vi "VGC50 Read Pressures.vi"(8 "error in (no error)":errorcluster, 11 "VGC50 In":T1={"serial settings"={"port"="", "baud rate"=115200}, "device information"={"type"="", "model number"="", "serial number"="", "firmware version"="", "hardware version"=""}, "VGC"=refnum, "Backing SP"={"mode"=0, "thresholds"={"lower"=0.0, "upper"=0.0}, "on"=FALSE}, "Chamber SP"={"mode"=1, "thresholds"={"lower"=0.0, "upper"=0.0}, "on"=FALSE}} {"Chamber SP"."thresholds"."upper" format="%#_5p"; "Chamber SP"."thresholds"."lower" format="%#_5p"; "Chamber SP"."mode" items=["off", "on", "channel 1", "channel 2", "channel 3"]; "Backing SP"."thresholds"."upper" format="%#_5p"; "Backing SP"."thresholds"."lower" format="%#_5p"; "Backing SP"."mode" items=["off", "on", "channel 1", "channel 2", "channel 3"]; "serial settings"."baud rate" items=["9600"=9600, "19200"=19200, "38400"=38400, "57600"=57600, "115200"=115200]}) -> (0 "error out":errorcluster, 1 "Chamber Pressure":dbl, 2 "Backing Pressure":dbl, 3 "VGC50 Out":T1={"serial settings"={"port"="", "baud rate"=115200}, "device information"={"type"="", "model number"="", "serial number"="", "firmware version"="", "hardware version"=""}, "VGC"=refnum, "Backing SP"={"mode"=0, "thresholds"={"lower"=0.0, "upper"=0.0}, "on"=FALSE}, "Chamber SP"={"mode"=1, "thresholds"={"lower"=0.0, "upper"=0.0}, "on"=FALSE}} {"Chamber SP"."thresholds"."upper" format="%#_5p"; "Chamber SP"."thresholds"."lower" format="%#_5p"; "Chamber SP"."mode" items=["off", "on", "channel 1", "channel 2", "channel 3"]; "Backing SP"."thresholds"."upper" format="%#_5p"; "Backing SP"."thresholds"."lower" format="%#_5p"; "Backing SP"."mode" items=["off", "on", "channel 1", "channel 2", "channel 3"]; "serial settings"."baud rate" items=["9600"=9600, "19200"=19200, "38400"=38400, "57600"=57600, "115200"=115200]}, 4 "Waveform Chart":waveform(dbl)[](graph))   [LabVIEW 2024]
uses:
  controls/VGC50.ctl
  <instrlib>/PL Inficon VGC/PL Inficon VGC.lvclass
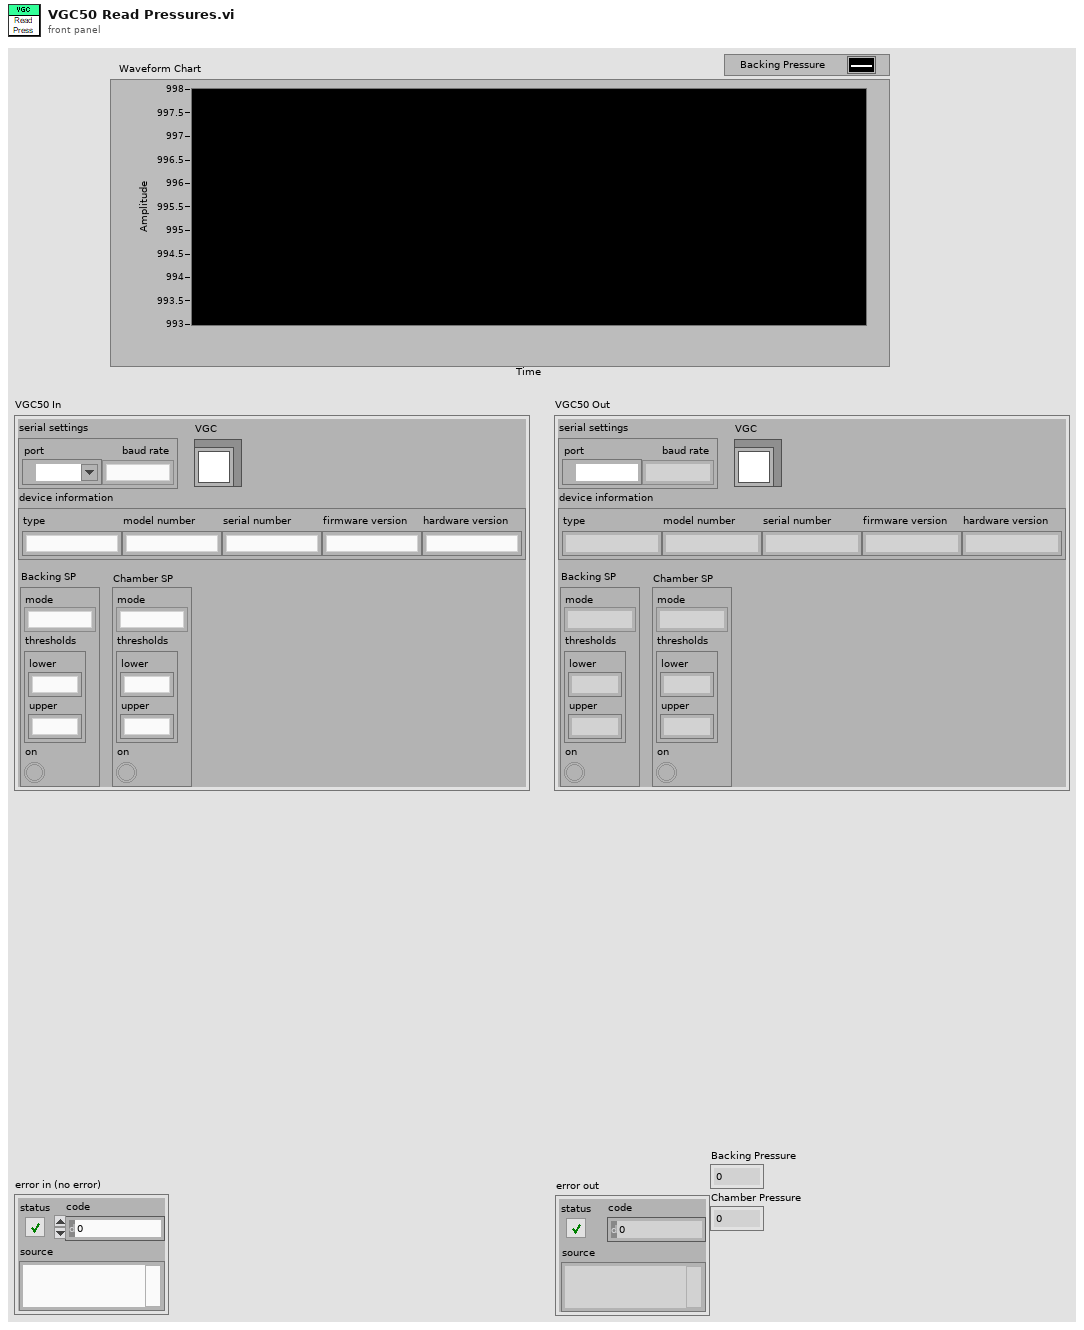
[diagram p1: front panel]
types:
  T1 = typedef "VGC50.ctl" = cluster{"serial settings":cluster{"port":refnum<visa-resource-name>, "baud rate":u32}, "device information":cluster{"type":string, "model number":string, "serial number":string, "firmware version":string, "hardware version":string}, "VGC":refnum<class "PL Inficon VGC.lvclass">, "Backing SP":cluster{"mode":u16, "thresholds":cluster{"lower":dbl, "upper":dbl}, "on":bool}, "Chamber SP":cluster{"mode":u16, "thresholds":cluster{"lower":dbl, "upper":dbl}, "on":bool}}
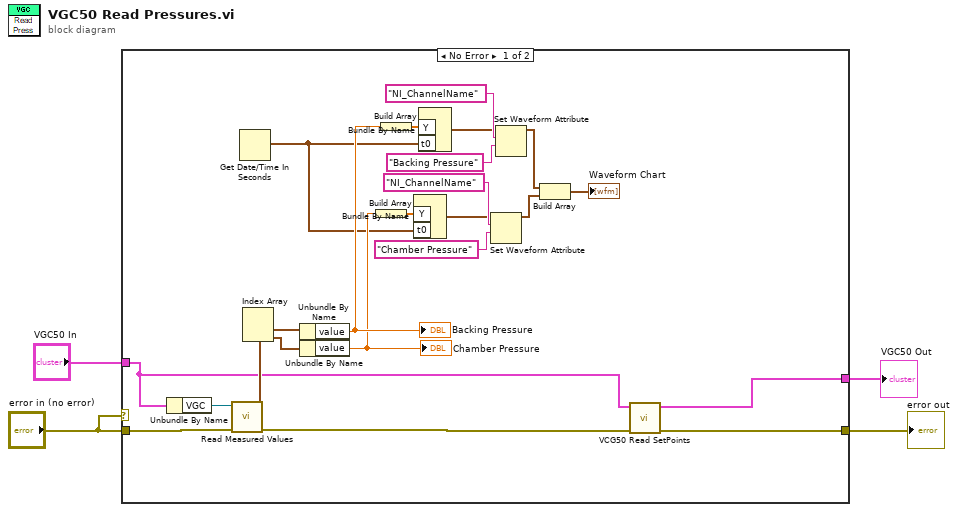
[diagram p0: block diagram]
diagram:
  n1 = case shown="No Error" "error in (no error)" {
    tunnel: "error in (no error)" -> [w21 w29]
    tunnel: "VGC50 In" -> [w23 w28]
    tunnel: [w19 w29] -> w2
    tunnel: [w22 w28] -> w1
    frame No Error {
      n2 = Unbundle By Name(w23) -> ("VGC"=w27:refnum<class "PL Inficon VGC.lvclass">)
      n3 = call <instrlib>:"Read Measured Values.vi"("error in (no error)"=w21, "VGC in"=w27) -> ("error out"=w20:errorcluster, "measured values"=w24:cluster{"status":u16, "value":dbl}[])  [unwired: 7 in, 1 out]
      n4 = Get Date/Time In Seconds() -> (seconds since 1Jan1904=w5:timestamp)
      n5 = Index Array(array=w24) -> (element #1=w26:cluster{"status":u16, "value":dbl}, element #2=w25:cluster{"status":u16, "value":dbl})  [unwired: 2 in]
      n6 = Unbundle By Name(w26) -> ("value"=w17:dbl)
      "Backing Pressure" <- w17
      n7 = Unbundle By Name(w25) -> ("value"=w9:dbl)
      "Chamber Pressure" <- w9
      n8 = Build Array(w9) -> (w13:dbl[])
      n9 = Build Array(w17) -> (w18:dbl[])
      n10 = Bundle By Name("Y"=w13, "t0"=w5) -> (w11:waveform(dbl))  [unwired: 1 in]
      n11 = Bundle By Name("Y"=w18, "t0"=w5) -> (w15:waveform(dbl))  [unwired: 1 in]
      n12 = Set Waveform Attribute(5:"Chamber Pressure" ("name"), 6:"NI_ChannelName" ("name"), 7:w11) -> (3:w7:waveform(dbl))  [unwired: 1 in, 2 out]
      n13 = Set Waveform Attribute(5:"Backing Pressure" ("name"), 6:"NI_ChannelName" ("name"), 7:w15) -> (3:w8:waveform(dbl))  [unwired: 1 in, 2 out]
      n14 = Build Array(w8, w7) -> (→"Waveform Chart":waveform(dbl)[])
      n15 = call "VCG50 Read SetPoints.vi"("error in (no error)"=w20, "VGC50 In"=w23) -> ("error out"=w19:errorcluster, "VGC50 Out"=w22:T1)  [unwired: 8 in]
    }
    frame Error {
    }
  }
  "VGC50 Out" <- w1
  "error out" <- w2
